vi "Teleop.vi"(10 "Match Info":T1={"Autonomous Elapsed Seconds"=0.0, "TeleOp Elapsed Seconds"=0.0, "Disabled Elapsed Seconds"=0.0, "Visited Autonomous"=FALSE, "Visited TeleOp"=FALSE, "Visited Disabled"=FALSE, "Autonomous Settings"={"Autonomous Style"=enum."Independent", "VI Refnum"=refnum}}, 11 "Call Context":T2) -> ()   [LabVIEW 2012]
doc: "This VI is called for each TeleOp packet received from the DS where the robot is not disabled. It is often used to read from the joysticks and update I/O or to update setpoints for timed control loops. It should complete and return within 20 milliseconds or it may miss DS packets."
uses:
  <vilib>/Rock Robotics/WPI/DriverStation/WPI_DriverStationDerivedRobotMode.ctl
  <vilib>/Rock Robotics/WPI/DriverStation/WPI_DriverStationMatch Info.ctl
  Robot Global Data.vi
  <vilib>/Rock Robotics/WPI/RobotDrive/WPI_RobotDriveArcadeDrive_Standard(NoSaturation).vi
  <vilib>/Rock Robotics/WPI/RobotDrive/WPI_RobotDriveGetSetRefNum.vi
  <vilib>/Rock Robotics/WPI/RobotDrive/WPI_RobotDriveMecanumDrive_Cartesian.vi
panel:
  in  "Slot 4":bool=TRUE
  in  "Slot 3":bool=TRUE
  in  "Slot 2":bool
  in  "Slot 1":bool
  out "Numeric 1":dbl(slide) scale=0.0..100.0
  out "Boolean 2":bool
  out "Boolean 1":bool
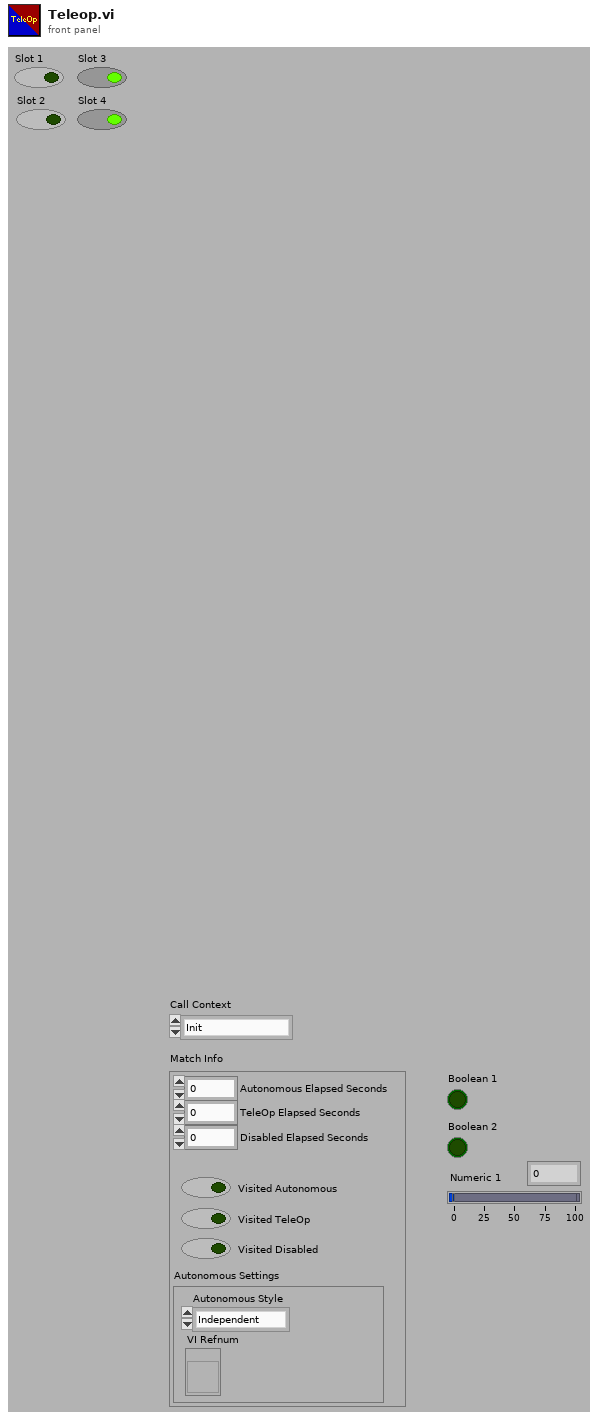
[diagram p1: front panel]
types:
  T1 = typedef "WPI_DriverStationMatch Info.ctl" = cluster{"Autonomous Elapsed Seconds":dbl, "TeleOp Elapsed Seconds":dbl, "Disabled Elapsed Seconds":dbl, "Visited Autonomous":bool, "Visited TeleOp":bool, "Visited Disabled":bool, "Autonomous Settings":cluster{"Autonomous Style":enum16{"Iterative", "Independent"}, "VI Refnum":refnum<vi>}}
  T2 = typedef "WPI_DriverStationDerivedRobotMode.ctl" = enum16{"Init", "Execute", "Stop"}
  T3 = typedef "WPI_RobotDriveDevRef.ctl" = cluster{"DevStatus":errorcluster, "Motors[]":T4[], "Square Inputs":bool, "Max Output":dbl, "Isochronous":bool}
  T4 = typedef "WPI_MotorControlDeviceRef.ctl" = cluster{"DeviceStatus":errorcluster, "Type":enum16{"PWM", "CAN"}, "PWM":cluster{"Digital Module":T5, "PWM Channel":T6, "DeadBand":T7}, "CAN":cluster{"Device Number":u8, "Control Mode":T8, "Semaphore":T9, "Max Vout":dbl}, "Invert":bool, "TransformRef":T10, "InvTransformRef":T10}
  T5 = typedef "FPGA_TypedefDigitalModule.ctl" = enum16{"Digital Module 1", "Digital Module 2"}
  T6 = typedef "FPGA_DIOPWMChannel.ctl" = enum8{"PWM 1", "PWM 2", "PWM 3", "PWM 4", "PWM 5", "PWM 6", "PWM 7", "PWM 8", "PWM 9", "PWM 10", "Invalid"}
  T7 = typedef "WPI_PWMDeadband.ctl" = cluster{"Name":string, "maxPositivePwm":i32, "minPositivePwm":i32, "centerPwm":i32, "maxNegativePwm":i32, "minNegativePwm":i32, "angularRange":u16}
  T8 = typedef "WPI_CANJaguar_ControlMode.ctl" = enum8{"Percent VBus", "Current", "Speed", "Position", "Voltage"}
  T9 = typedef "Semaphore RefNum" = refnum<k1>
  T10 = typedef "WPI_PWMTransform_ConPane.ctl" = refnum<vi>
  T11 = typedef "WPI_ServoDeviceRef.ctl" = cluster{"DeviceStatus":errorcluster, "Digital Module":T5, "PWM Channel":T6, "DeadBand":T7}
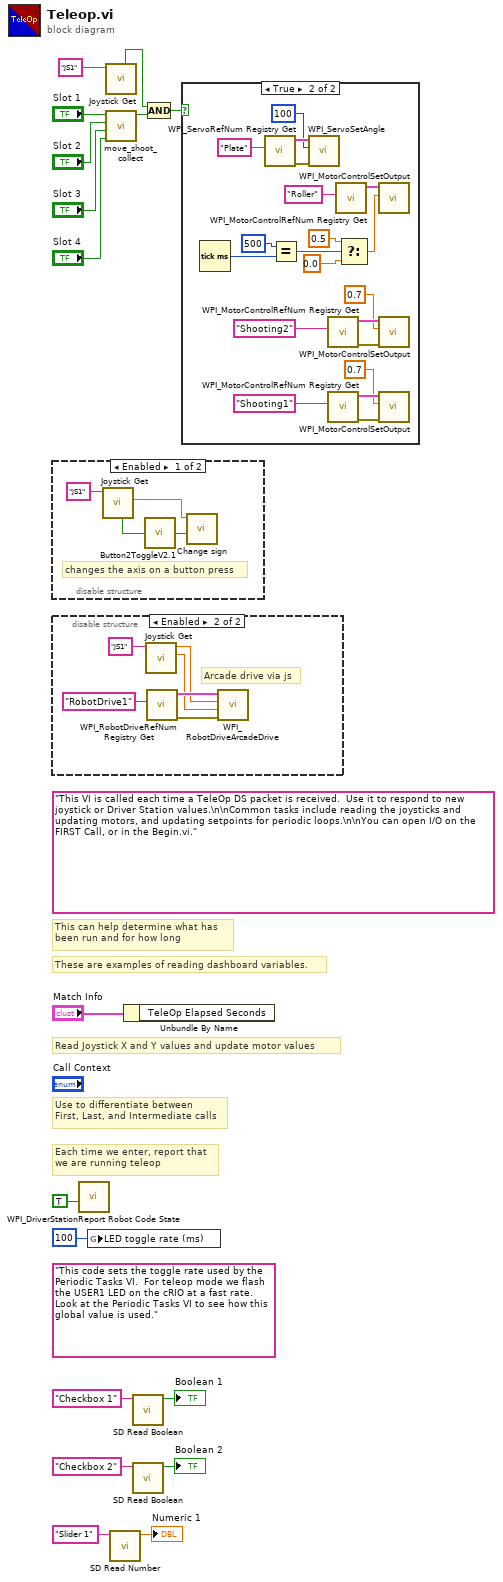
[diagram p0: block diagram]
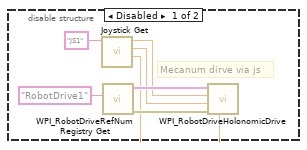
[diagram p4: hidden frame]
diagram:
  (unwired) "This code sets the toggle rate used by the Periodic Tasks VI.  For teleop mode we flash the USER1 LED on the cRIO at a fast rate.  Look at the Periodic Tasks VI to see how this global value is used."
  (unwired) "This VI is called each time a TeleOp DS packet is received.  Use it to respond to new joystick or Driver Station values.\n\nCommon tasks include reading the joysticks and updating motors, and updating setpoints for periodic loops.\n\nYou can open I/O on the FIRST Call, or in the Begin.vi."
  # "These are examples of reading dashboard variables."
  # "Each time we enter, report that\nwe are running teleop"
  # "Use to differentiate between\nFirst, Last, and Intermediate calls"
  # "This can help determine what has\nbeen run and for how long"
  # "Read Joystick X and Y values and update motor values"
  n1 = disable-structure shown="Enabled" {
    frame Enabled {
      # "changes the axis on a button press"
      n2 = call "Joystick Get.vi"("Js name"="JS1" ("refnum name")) -> ("axis 2 (y)"=w20:dbl, "Button 12"=w19:bool)  [unwired: 5 in, 4 out]
      n3 = call "Button2ToggleV2.1.vi"("a"=w19) -> ("Result(clone)"=w18:bool)
      n4 = call "Change sign.vi"("Boolean"=w18, "x"=w20) -> ()  [unwired: 8 in, 2 out]
    }
    frame Disabled {
    }
  }
  n5 = disable-structure shown="Enabled" {
    frame Disabled {
      # "Mecanum dirve via js"
      n6 = call "Joystick Get.vi"("Js name"="JS1" ("refnum name")) -> ("axis 3 (throttle)"=w22:dbl, "axis 2 (y)"=w23:dbl, "axis 1 (x)"=w24:dbl)  [unwired: 5 in, 3 out]
      n7 = call <vilib>:"WPI_RobotDriveRefNum Registry Get.vi"("refnum name"="RobotDrive1") -> ("error out"=w28:errorcluster, "RobotDriveDevRef"=w27:T3)  [unwired: 9 in]
      n8 = call-poly <vilib>:"WPI_RobotDriveHolonomicDrive.vi"("Rotation"=w22, "error in (no error)"=w28, "Y"=w23, "X"=w24, "RobotDriveDevRef"=w27) -> ()  [unwired: 4 in, 3 out]
    }
    frame Enabled {
      # "Arcade drive via js"
      n9 = call "Joystick Get.vi"("Js name"="JS1" ("refnum name")) -> ("axis 2 (y)"=w29:dbl, "axis 1 (x)"=w30:dbl)  [unwired: 5 in, 4 out]
      n10 = call <vilib>:"WPI_RobotDriveRefNum Registry Get.vi"("refnum name"="RobotDrive1") -> ("error out"=w32:errorcluster, "RobotDriveDevRef"=w31:T3)  [unwired: 9 in]
      n11 = call-poly <vilib>:"WPI_RobotDriveArcadeDrive.vi"("error in (no error)"=w32, "Y axis value"=w29, "X axis value"=w30, "RobotDriveDevRef"=w31) -> ()  [unwired: 5 in, 3 out]
    }
  }
  n12 = call <vilib>:"WPI_DriverStationReport Robot Code State.vi"("TeleOp"=TRUE ("Autonomous")) -> ()  [unwired: 10 in, 1 out]
  n13 = global write "Robot Global Data.vi" "LED toggle rate (ms)"(u32 100 ("LED ms toggle rate")) -> ()
  n14 = call "Joystick Get.vi"("Js name"="JS1" ("refnum name")) -> ("Button 1"=w3:bool)  [unwired: 5 in, 5 out]
  n15 = call "move_shoot_collect.vi"("Slot 4"="Slot 4", "Slot 3"="Slot 3", "Slot 2"="Slot 2", "Slot 1"="Slot 1") -> ("Shoot"=w2:bool)  [unwired: 3 in, 4 out]
  n16 = call <vilib>:"SD Read Number.vi"("Name"="Slider 1" ("refnum name")) -> ("Numeric"=→"Numeric 1":dbl)  [unwired: 8 in, 2 out]
  n17 = Unbundle By Name("Match Info") -> ()  [unwired: 1 out]
  n18 = call <vilib>:"SD Read Boolean.vi"("Name"="Checkbox 1" ("refnum name")) -> ("Boolean"=→"Boolean 1":bool)  [unwired: 8 in, 2 out]
  n19 = call <vilib>:"SD Read Boolean.vi"("Name"="Checkbox 2" ("refnum name")) -> ("Boolean"=→"Boolean 2":bool)  [unwired: 8 in, 2 out]
  n20 = Compound Arithmetic op=AND(w3, w2) -> (w1:bool)
  n21 = case shown="True" w1 {
    frame False {
    }
    frame True {
      n22 = Tick Count (ms)() -> (millisecond timer value=w49:u32)
      n23 = call <vilib>:"WPI_ServoRefNum Registry Get.vi"("refnum name"="Plate") -> ("error out"=w54:errorcluster, "ServoDeviceRef"=w53:T11)  [unwired: 9 in]
      n24 = Equal?(x=u32 500, y=w49) -> (x = y?=w48:bool)
      n25 = call <vilib>:"WPI_ServoSetAngle.vi"("error in (no error)"=w54, "Angle"=100, "ServoDeviceRef"=w53) -> ()  [unwired: 7 in, 2 out]
      n26 = call <vilib>:"WPI_MotorControlRefNum Registry Get.vi"("refnum name"="Shooting2") -> ("error out"=w38:errorcluster, "MotorControlDevRef"=w37:T4)  [unwired: 9 in]
      n27 = call <vilib>:"WPI_MotorControlRefNum Registry Get.vi"("refnum name"="Shooting1") -> ("error out"=w42:errorcluster, "MotorControlDevRef"=w41:T4)  [unwired: 9 in]
      n28 = call <vilib>:"WPI_MotorControlRefNum Registry Get.vi"("refnum name"="Roller") -> ("MotorControlDevRef"=w45:T4)  [unwired: 9 in, 1 out]
      n29 = Select(t=0.5, s=w48, f=0.0) -> (s? t:f=w43:dbl)
      n30 = call <vilib>:"WPI_MotorControlSetOutput.vi"("Output"=w43, "MotorControlDevRef"=w45) -> ()  [unwired: 7 in, 3 out]
      n31 = call <vilib>:"WPI_MotorControlSetOutput.vi"("error in (no error)"=w38, "Output"=0.7, "MotorControlDevRef"=w37) -> ()  [unwired: 6 in, 3 out]
      n32 = call <vilib>:"WPI_MotorControlSetOutput.vi"("error in (no error)"=w42, "Output"=0.7, "MotorControlDevRef"=w41) -> ()  [unwired: 6 in, 3 out]
    }
  }
